vi "画面中心画+7500相机.vi"(11 "引用句柄输入":T1) -> (3 "引用句柄输出":T1)   [LabVIEW 2014]
uses:
  <vilib>/vision/Image Controls.llb/IMAQ Image.ctl
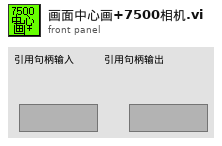
[diagram p1: front panel]
types:
  T1 = typedef "IMAQ Image.ctl" = refnum<image>
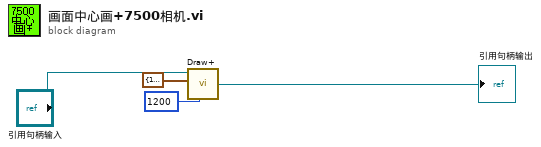
[diagram p0: block diagram]
diagram:
  n1 = call "Draw+.vi"("Width"=1200, "input cluster"=cluster{"P_X":i32, "P_Y":i32} {"P_X"=1224, "P_Y"=1024}, "Image In"="引用句柄输入") -> ("Image Out"=→"引用句柄输出":T1)  [unwired: 3 in]
